vi "Read Channel info.vi"(8 "error in":errorcluster, 11 "channel in":refnum<class "channel node.lvclass">) -> (0 "error out":errorcluster, 2 "channel info":T1, 3 "channel out":refnum<class "channel node.lvclass">)   [LabVIEW 2013, in "channel node.lvclass"]
uses:
  channel node.lvclass
  channel configuration/ChannelData.ctl
  channel node.lvclass/channel node.ctl
  channel configuration/channel configuration.lvclass/channel configuration.ctl
  channel configuration/channel configuration.lvclass
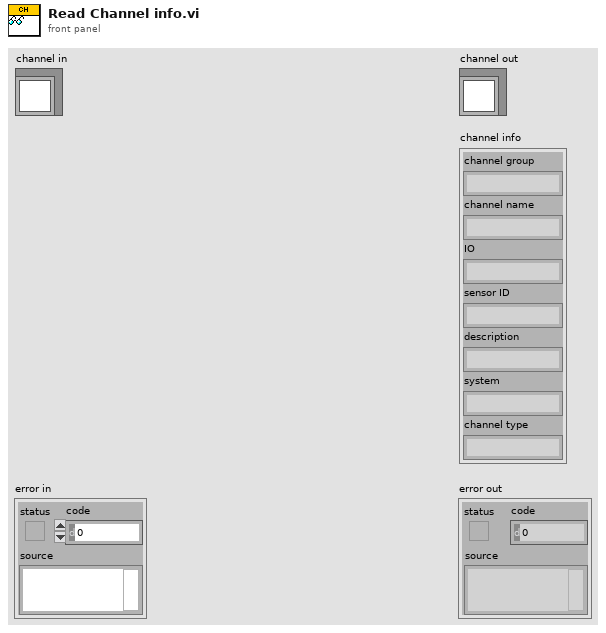
[diagram p1: front panel]
types:
  T1 = typedef "channel configuration.lvclass/ChannelData.ctl" = cluster{"channel group":string, "channel name":string, "IO":string, "sensor ID":string, "description":string, "system":string, "channel type":string}
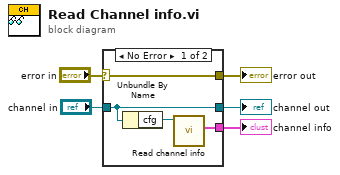
[diagram p0: block diagram]
diagram:
  n1 = case shown="No Error" "error in" {
    selector: "error in" -> [w9 w10]
    tunnel: [w9 w10] -> w4
    tunnel: [w8 w11] -> w2
    tunnel: "channel in" -> [w8 w11]
    tunnel: [w6 _] -> w1
    frame No Error {
      n2 = Unbundle By Name(w8) -> ("cfg"=w7:refnum<class "channel configuration.lvclass">)
      n3 = call "Read channel info.vi"("channel config object in"=w7) -> ("channel"=w6:T1)  [unwired: 8 in, 2 out]
    }
    frame Error {
    }
  }
  "error out" <- w4
  "channel out" <- w2
  "channel info" <- w1
